vi "Locate edges.vi"(6 "Seen last value":bool, 9 "Last value":i32, 10 "First value":i32, 11 "Values":i32[](array[numeric])) -> (1 "Ending edges":i32[](array[numeric]), 2 "Seen last value 2":bool, 3 "Starting edges":i32[](array[numeric]), 4 "Seen last value out":bool)   [LabVIEW 2019]
panel:
  out "Numeric Control":i32
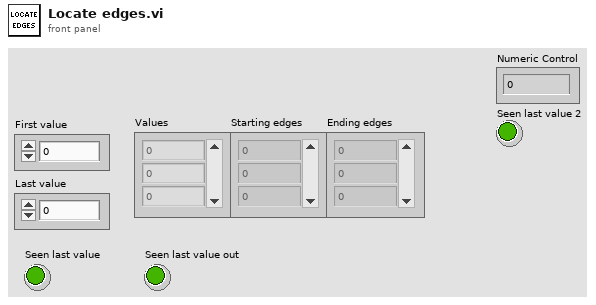
[diagram p1: front panel]
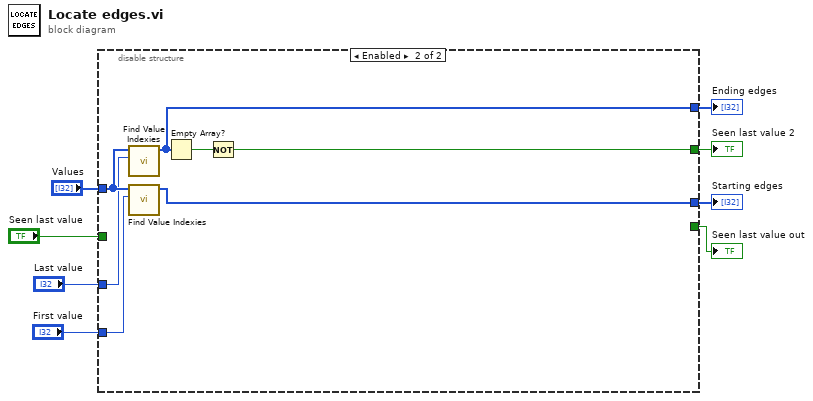
[diagram p0: block diagram]
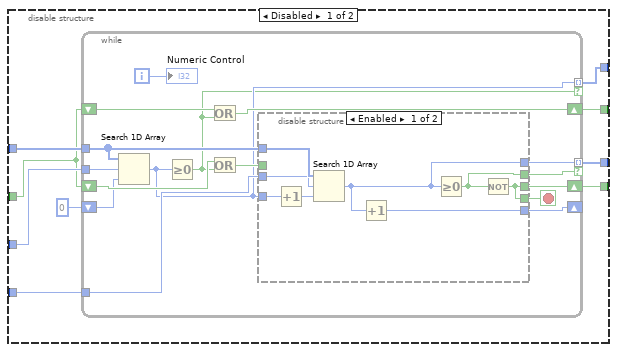
[diagram p2: hidden frame]
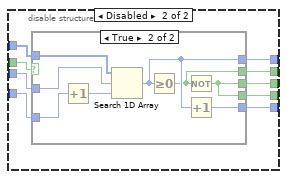
[diagram p3: hidden frame]
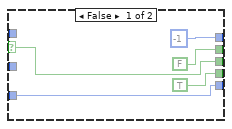
[diagram p4: hidden frame]
diagram:
  n1 = disable-structure shown="Enabled" {
    disable-tunnel: "First value" -> [w16 w70]
    disable-tunnel: "Last value" -> [w15 w67]
    disable-tunnel: "Values" -> [w14 w68]
    disable-tunnel: [w13 w69] -> w5
    disable-tunnel: [w12 _] -> w4
    disable-tunnel: "Seen last value" -> [w11 _]
    disable-tunnel: [w10 w64] -> w2
    disable-tunnel: [w9 w66] -> w1
    frame Disabled {
      n2 = while {
        tunnel: w15 -> [w33]
        tunnel: w14 -> [w30]
        tunnel: w16 -> [w29]
        shift-right: [w24] -> w12
        shift-left: w11 -> [w32]
        tunnel: [w28] -> w13 mode=indexing if=w27
        shift-right: [w25] -> _
        shift-left: 0 -> [w26]
        shift-right: [w20] -> w10
        shift-left: w11 -> [w21]
        tunnel: [w19] -> w9 mode=indexing if=w18
        i -> [w22]
        stop <- w23 stop-if-true
        n3 = Search 1D Array(1D array=w30, element=w33, start index (0)=w26) -> (index of element=w19:i32)
        n4 = Greater Or Equal To 0?(x=w19) -> (x >= 0?=w18:bool)
        n5 = Or(x=w21, y=w18) -> (x .or. y?=w20:bool)
        n6 = Or(x=w32, y=w18) -> (x .or. y?=w31:bool)
        n7 = disable-structure shown="Enabled" {
          disable-tunnel: w31 -> [_ w50]
          disable-tunnel: w30 -> [w41 w49]
          disable-tunnel: w29 -> [w40 w48]
          disable-tunnel: [w39 w47] -> w28
          disable-tunnel: [w38 w46] -> w27
          disable-tunnel: [w37 w45] -> w25
          disable-tunnel: [w36 w44] -> w24
          disable-tunnel: [w36 w43] -> w23
          disable-tunnel: w19 -> [w35 w42]
          frame Enabled {
            n8 = Increment(x=w35) -> (x+1=w34:i32)
            n9 = Search 1D Array(1D array=w41, element=w40, start index (0)=w34) -> (index of element=w39:i32)
            n10 = Increment(x=w39) -> (x+1=w37:i32)
            n11 = Greater Or Equal To 0?(x=w39) -> (x >= 0?=w38:bool)
            n12 = Not(x=w38) -> (.not. x?=w36:bool)
          }
          frame Disabled {
            n13 = case shown="True" w50 {
              selector: w50 -> [w52 _]
              tunnel: w49 -> [_ w63]
              tunnel: w42 -> [w53 w61]
              tunnel: w48 -> [_ w60]
              tunnel: [-1 ("index of element") w58] -> w47
              tunnel: [FALSE w57] -> w46
              tunnel: [w53 w59] -> w45
              tunnel: [w52 w56] -> w44
              tunnel: [TRUE w56] -> w43
              frame False {
              }
              frame True {
                n14 = Increment(x=w61) -> (x+1=w62:i32)
                n15 = Search 1D Array(1D array=w63, element=w60, start index (0)=w62) -> (index of element=w58:i32)
                n16 = Greater Or Equal To 0?(x=w58) -> (x >= 0?=w57:bool)
                n17 = Not(x=w57) -> (.not. x?=w56:bool)
                n18 = Increment(x=w58) -> (x+1=w59:i32)
              }
            }
          }
        }
        "Numeric Control" <- w22
      }
    }
    frame Enabled {
      n19 = call "Find Value Indexies.vi"("Value"=w67, "Array"=w68) -> ("Value indexies"=w66:i32[])  [unwired: 9 in]
      n20 = call "Find Value Indexies.vi"("Value"=w70, "Array"=w68) -> ("Value indexies"=w69:i32[])  [unwired: 9 in]
      n21 = Empty Array?(array=w66) -> (empty?=w65:bool)
      n22 = Not(x=w65) -> (.not. x?=w64:bool)
    }
  }
  "Seen last value out" <- w4
  "Starting edges" <- w5
  "Seen last value 2" <- w2
  "Ending edges" <- w1
